vi "OnValueChange_leftJoy.vi"(8 "error in (no error)":errorcluster, 9 "direction":T1, 11 "Game in":refnum<class "Game.lvclass">) -> (0 "error out":errorcluster, 3 "Game out":refnum<class "Game.lvclass">)   [LabVIEW 2019, in "RT_Game.lvlib" / "Game.lvclass"]
uses:
  Game.lvclass
  Engine/JoystickDir.ctl
  Engine/Engine.lvclass
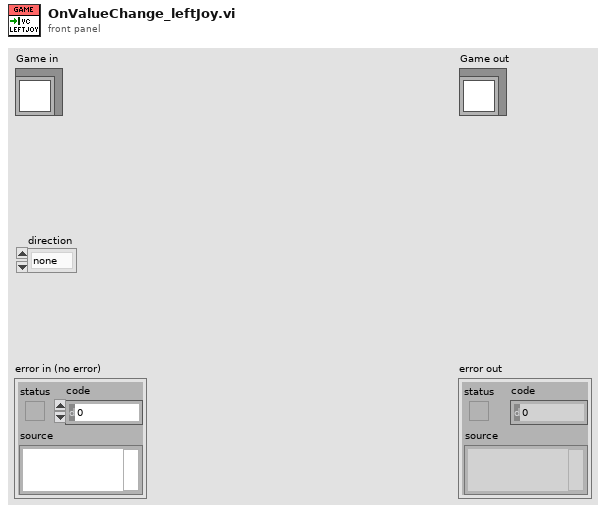
[diagram p1: front panel]
types:
  T1 = typedef "RT_Game.lvlib/Engine.lvclass/JoystickDir.ctl" = enum16{"none", "left", "right", "leftrightUNUSED", "up", "upLeft", "upRight", "upLeftRightUNUSED", "down", "downLeft", "downRight", "downLeftRightUNUSED", "upDownUNUSED", "upDownLeftUNUSED", "upDownRightUNUSED", "upDownRightLeftUNUSED"}
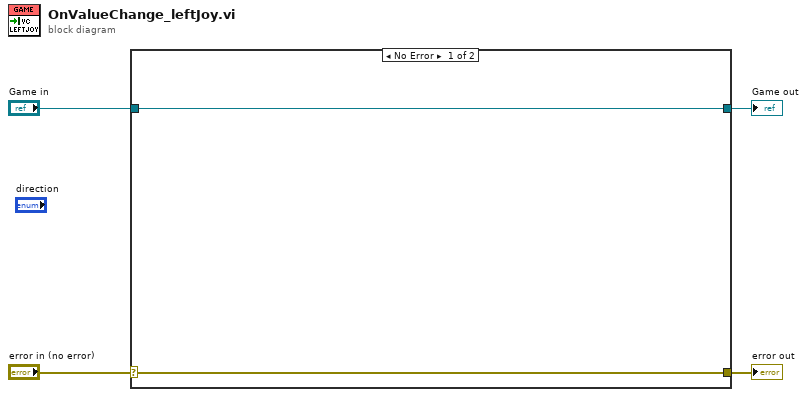
[diagram p0: block diagram]
diagram:
  n1 = case shown="No Error" "error in (no error)" {
    selector: "error in (no error)" -> [w5 w8]
    tunnel: [w5 w8] -> w3
    tunnel: [w6 w7] -> w1
    tunnel: "Game in" -> [w6 w7]
    frame No Error {
    }
    frame Error {
    }
  }
  "error out" <- w3
  "Game out" <- w1
